vi "Test_WriteValue_TransportClosed_WriteError.vi"(8 "error in (no error)":errorcluster, 11 "TestCase in":refnum<class "TestNotifierTransport.lvclass">) -> (0 "error out":errorcluster, 3 "TestCase out":refnum<class "TestNotifierTransport.lvclass">)   [LabVIEW 2017, in "TestNotifierTransport.lvclass"]
uses:
  TestNotifierTransport.lvclass
  Source/Concrete/NotifierTransport/NotifierTransport.lvclass/NotifierTransport.ctl
  Source/Concrete/NotifierTransport/NotifierTransport.lvclass
  C:/Git/composed-transport/Source/ITransport/ITransport.lvclass
  Source/ITransport/ITransport.lvclass
panel:
  out "Return Error":errorcluster
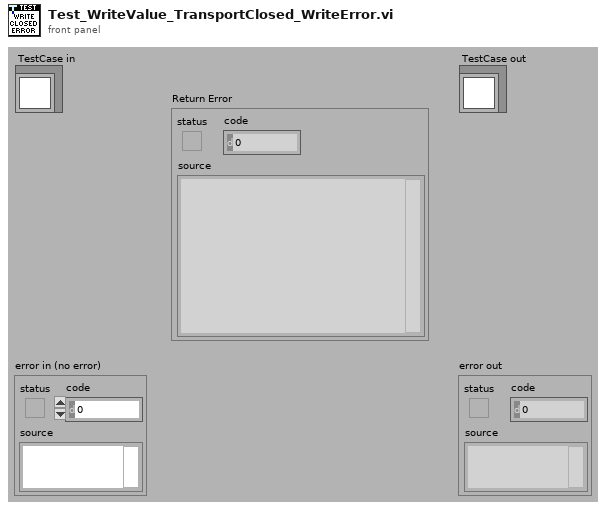
[diagram p1: front panel]
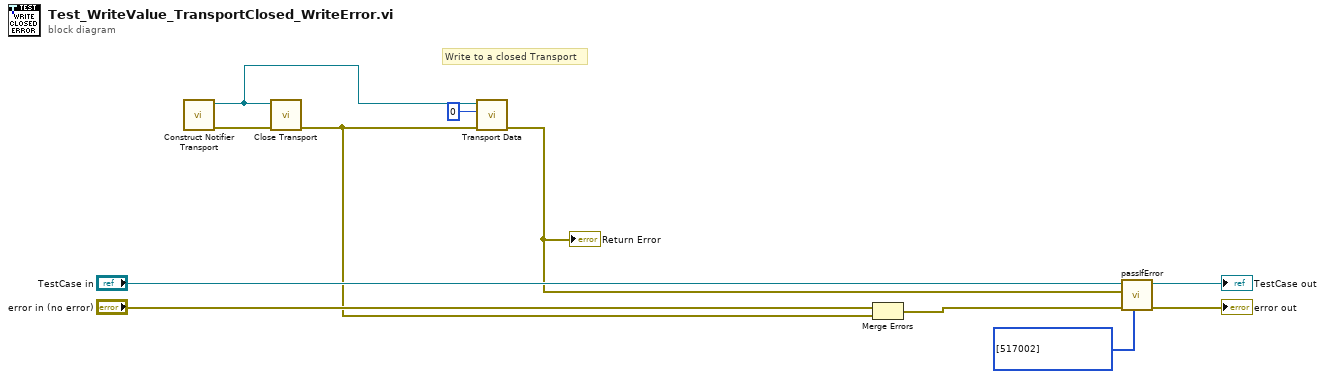
[diagram p0: block diagram]
diagram:
  # "Write to a closed Transport"
  n1 = call "Construct Notifier Transport.vi"() -> ("error out"=w3:errorcluster, "NotifierTransport"=w2:refnum<class "NotifierTransport.lvclass">)  [unwired: 10 in]
  n2 = call-dynamic "Close Transport.vi"("error in (no error)"=w3, "NotifierTransport"=w2) -> ("error out"=w1:errorcluster)  [unwired: 9 in]
  n3 = call "Transport Data.vi"("error in (no error)"=w1, "Value"=0, "ITransport in"=w2) -> ("error out"=w5:errorcluster)  [unwired: 7 in, 1 out]
  "Return Error" <- w5
  n4 = Merge Errors("error in (no error)", w1) -> (w6:errorcluster)
  n5 = call-dynamic "passIfError.vi"("passing error codes (default = any error code)"=i32[] [517002], "error in (no error)"=w6, "error"=w5, "TestCase in"="TestCase in") -> ("error out"=→"error out":errorcluster, "TestCase out"=→"TestCase out":refnum<class "TestNotifierTransport.lvclass">)  [unwired: 6 in]
